vi "U3 Create PWM16 Lists.vi"() -> (1 "Period List":dbl[][](array[numeric]) format="%.6f", 2 "Frequency List":dbl[][](array[numeric]) format="%.6f")   [LabVIEW 2021]
panel:
  # "Creates 2D arrays which are lists of all the frequency/period\noptions for PWM16 timer mode 0.\n\nFrequency/Period, Base Clock, Divisor"
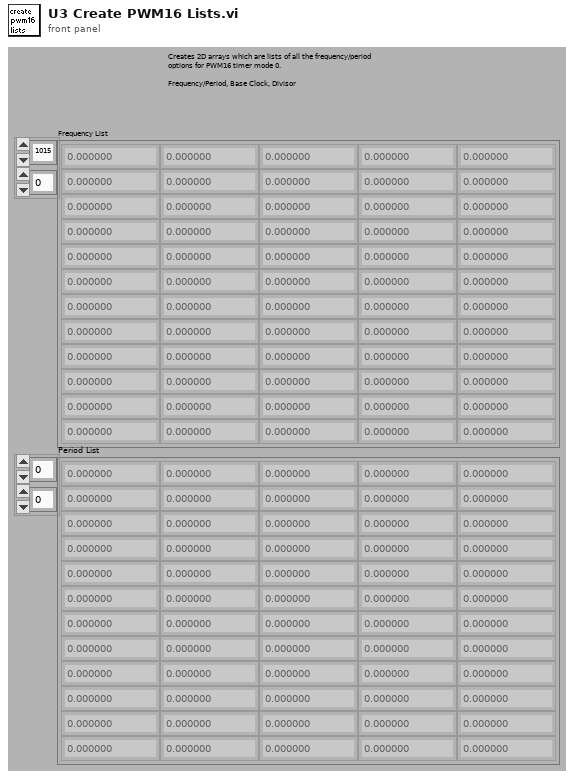
[diagram p1: front panel]
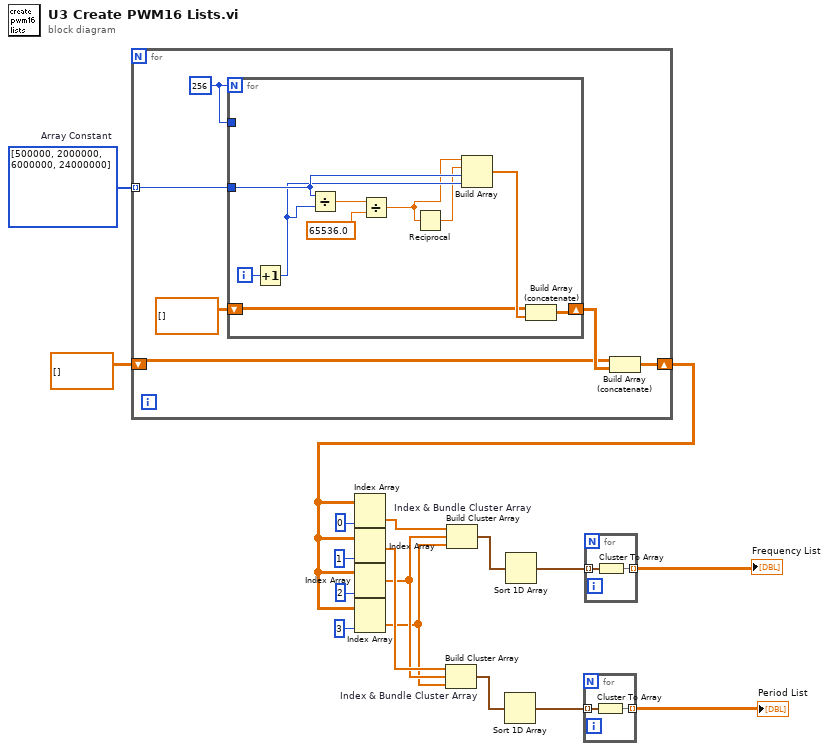
[diagram p0: block diagram]
diagram:
  w15 = i32[] [500000, 2000000, 6000000, 24000000]  # Array Constant
  n1 = for {
    tunnel: w15 -> [w23] mode=indexing
    shift-right: [w19] -> w7
    shift-left: dbl[][] [] -> [w20]
    w22 = 256
    n2 = for {
      N: w22 -> [_]
      tunnel: w23 -> [w33]
      tunnel: w22 -> [_]
      shift-right: [w28] -> w21
      shift-left: dbl[][] [] -> [w29]
      i -> [w32]
      n3 = Increment(x=w32) -> (x+1=w31:i32)
      n4 = Divide(x=w33, y=w31) -> (x/y=w25:dbl)
      n5 = Divide(x=w25, y=65536.0) -> (x/y=w24:dbl)
      n6 = Reciprocal(x=w24) -> (1/x=w27:dbl)
      n7 = Build Array(w24, w27, w33, w31) -> (w30:dbl[])
      n8 = Build Array (concatenate)(w29, w30) -> (w28:dbl[][])
    }
    n9 = Build Array (concatenate)(w20, w21) -> (w19:dbl[][])
  }
  n10 = Index Array(array=w7, index (col)=0) -> (element=w13:dbl[])  [unwired: 1 in]
  n11 = Index Array(array=w7, index (col)=1) -> (element=w3:dbl[])  [unwired: 1 in]
  n12 = Index Array(array=w7, index (col)=2) -> (element=w2:dbl[])  [unwired: 1 in]
  n13 = Index Array(array=w7, index (col)=3) -> (element=w1:dbl[])  [unwired: 1 in]
  n14 = Build Cluster Array "Index & Bundle Cluster Array"(w3, w2, w1) -> (w4:cluster{dbl, dbl, dbl}[])
  n15 = Build Cluster Array "Index & Bundle Cluster Array"(w13, w2, w1) -> (w12:cluster{dbl, dbl, dbl}[])
  n16 = Sort 1D Array(array=w4) -> (sorted array=w5:cluster{dbl, dbl, dbl}[])
  n17 = Sort 1D Array(array=w12) -> (sorted array=w11:cluster{dbl, dbl, dbl}[])
  n18 = for {
    tunnel: w5 -> [w35] mode=indexing
    tunnel: [w34] -> w16 mode=indexing
    n19 = Cluster To Array(cluster=w35) -> (array=w34:dbl[])
  }
  "Period List" <- w16
  n20 = for {
    tunnel: w11 -> [w37] mode=indexing
    tunnel: [w36] -> w17 mode=indexing
    n21 = Cluster To Array(cluster=w37) -> (array=w36:dbl[])
  }
  "Frequency List" <- w17
